vi "Sub Exit.vi"(8 "error in (no error)":errorcluster, 11 "LF2R IDE in":refnum<class "Main Panel.lvclass">) -> (0 "error out":errorcluster, 3 "LF2R IDE out":refnum<class "Main Panel.lvclass">)   [LabVIEW 2018, in "Main Panel.lvlib" / "Main Panel.lvclass"]
uses:
  Main Panel.lvclass
  C:/Program Files (x86)/National Instruments/LabVIEW 2018/vi.lib/ActorFramework/Actor/Actor.lvclass
  Main Panel.lvclass/Main Panel.ctl
  <vilib>/ActorFramework/Actor/Actor.lvclass/Actor.ctl
  <vilib>/ActorFramework/Message Enqueuer/Message Enqueuer.lvclass/Message Enqueuer.ctl
  <vilib>/ActorFramework/Message Enqueuer/Enqueue.vi
  <vilib>/ActorFramework/Message Enqueuer/Init from Existing Queue.vi
  <vilib>/ActorFramework/Stop Msg/Stop Msg.lvclass
  C:/Program Files (x86)/National Instruments/LabVIEW 2018/vi.lib/ActorFramework/Message/Message.lvclass
  <vilib>/ActorFramework/Message Priority Queue/Priority Enqueue.vi
  <vilib>/ActorFramework/Message Enqueuer/Message Enqueuer.lvclass
  <vilib>/ActorFramework/Actor/Actor.lvclass
  ScintillaNET/ScintillaNET.lvclass
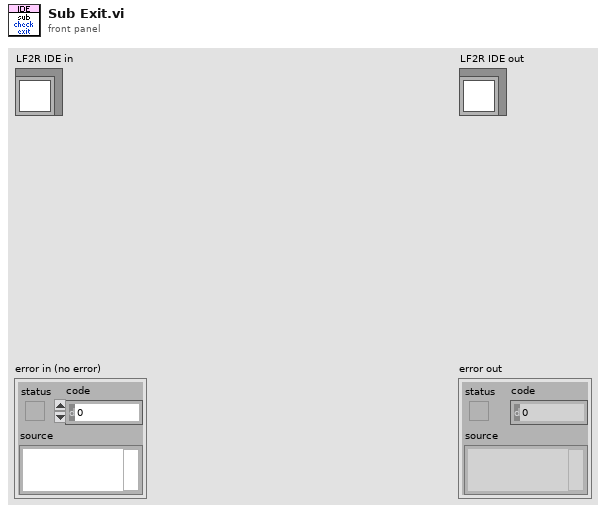
[diagram p1: front panel]
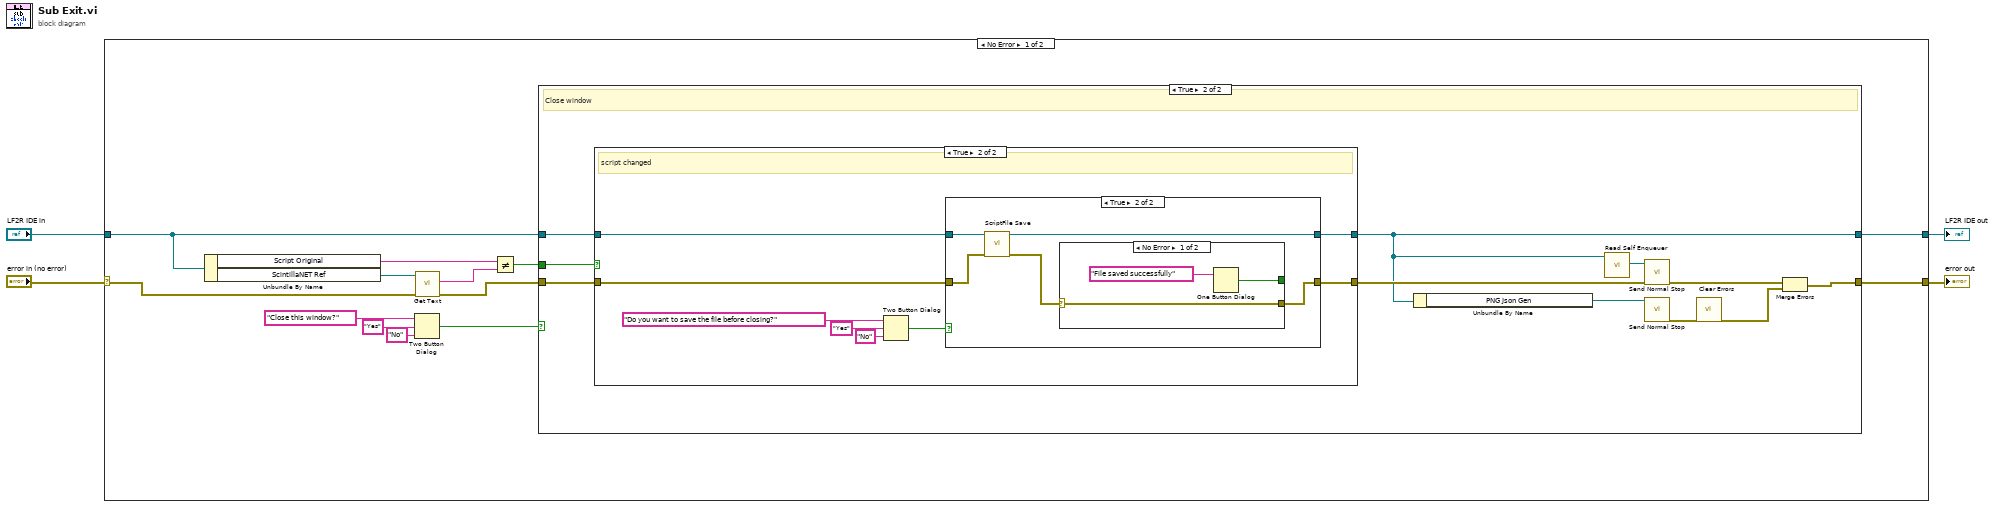
[diagram p0: block diagram]
diagram:
  n1 = case shown="No Error" "error in (no error)" {
    selector: "error in (no error)" -> [w6 w53]
    tunnel: [w10 w53] -> w3
    tunnel: [w11 w52] -> w1
    tunnel: "LF2R IDE in" -> [w12 w52]
    frame No Error {
      n2 = Unbundle By Name(w12) -> ("Script Original"=w14:string, "ScintillaNET Ref"=w9:refnum<class "ScintillaNET.lvclass">)
      n3 = Two Button Dialog(message="Close this window?", 1:"No" ("F button name (\"Cancel\")"), 2:"Yes" ("T button name (\"OK\")")) -> (T button?=w5:bool)
      n4 = call "Get Text.vi"("error in (no error)"=w6, "ScintillaNET in"=w9) -> ("error out"=w7:errorcluster, "Text"=w8:string)  [unwired: 7 in, 1 out]
      n5 = Not Equal?(x=w14, y=w8) -> (x != y?=w13:bool)
      n6 = case shown="True" w5 {
        tunnel: w13 -> [_ w30]
        tunnel: w12 -> [w19 w29]
        tunnel: [w19 w25] -> w11
        tunnel: [w18 w21] -> w10
        tunnel: w7 -> [w18 w27]
        frame False {
          # "Cancel"
        }
        frame True {
          # "Close window"
          n7 = case shown="True" w30 {
            tunnel: w29 -> [w32 w36]
            tunnel: w27 -> [w31 w35]
            tunnel: [w32 w34] -> w25
            tunnel: [w31 w33] -> w28
            frame False {
            }
            frame True {
              # "script changed"
              n8 = Two Button Dialog(message="Do you want to save the file before closing?", 1:"No" ("F button name (\"Cancel\")"), 2:"Yes" ("T button name (\"OK\")")) -> (T button?=w37:bool)
              n9 = case shown="True" w37 {
                tunnel: w36 -> [w41 w47]
                tunnel: w35 -> [w42 w46]
                tunnel: [w41 w45] -> w34
                tunnel: [w42 w43] -> w33
                frame False {
                }
                frame True {
                  n10 = call "ScriptFile Save.vi"("error in (no error)"=w46, "LF2R IDE in"=w47) -> ("error out"=w44:errorcluster, "LF2R IDE out"=w45:refnum<class "Main Panel.lvclass">)  [unwired: 7 in, 1 out]
                  n11 = case shown="No Error" w44 {
                    selector: w44 -> [w49 w51]
                    tunnel: [w49 w51] -> w43
                    tunnel: [w48 _] -> _
                    frame No Error {
                      n12 = One Button Dialog(message="File saved successfully") -> (true=w48:bool)  [unwired: 1 in]
                    }
                    frame Error {
                    }
                  }
                }
              }
            }
          }
          n13 = Unbundle By Name(w25) -> ("PNG Json Gen"=w24:refnum<class "Message Enqueuer.lvclass">)
          n14 = call <vilib>:"Read Self Enqueuer.vi"("Actor"=w25) -> ("Self Enqueuer"=w26:refnum<class "Message Enqueuer.lvclass">)  [unwired: 10 in]
          n15 = call <vilib>:"Send Normal Stop.vi"("error in (no error)"=w28, "Message Enqueuer"=w26) -> ("error out"=w22:errorcluster)  [unwired: 9 in]
          n16 = call <vilib>:"Send Normal Stop.vi"("Message Enqueuer"=w24) -> ("error out"=w23:errorcluster)  [unwired: 10 in]
          n17 = call <vilib>:"Clear Errors.vi"("error in (no error)"=w23) -> ("error out"=w20:errorcluster)  [unwired: 5 in, 1 out]
          n18 = Merge Errors(w22, w20) -> (w21:errorcluster)
        }
      }
    }
    frame Error {
    }
  }
  "error out" <- w3
  "LF2R IDE out" <- w1
